vi "Set 2D Next Vector_IS_BAK.vi"(0 "Coordinate System":u16(ring) items=["Cartesian", "Polar"], 1 "Magnetic Field Units":u16(ring) items=["kG", "Tesla"], 2 "Input Vector":string[](array[string]), 3 "User defined Ramp Rate (T/min)":dbl format="%.3f", 4 "Magnitude Limit (kG)":dbl format="%.3f", 5 "Y-Axis Communications Config":T3={"GPIB address"=22, "GPIB bus"=0, "connection ID"=refnum, "IP"="192.168.2.200", "Active Comm Interface"=0, "Serial Port"="", "Programmer Type"=0} {"Programmer Type" items=["Model 430", "Model 420"]; "Active Comm Interface" items=["TCP/IP (Model 430 Only)", "RS232", "IEEE488"]}, 6 "Tolerance (mT)":dbl=0.2 format="%#_13g", 7 "Z-Axis Communications Config":T3={"GPIB address"=22, "GPIB bus"=0, "connection ID"=refnum, "IP"="192.168.2.200", "Active Comm Interface"=0, "Serial Port"="", "Programmer Type"=0} {"Programmer Type" items=["Model 430", "Model 420"]; "Active Comm Interface" items=["TCP/IP (Model 430 Only)", "RS232", "IEEE488"]}, 9 "Tolerance (deg)":dbl=0.1 format="%#_13g", 10 "User defined Ramp Rate (T/min)":bool, 13 "Max Ramp Rate - Y Axis (A/s)":dbl format="%.3f", 14 "error in":T2, 15 "Max Ramp Rate - Z Axis (A/s)":dbl format="%.3f") -> (8 "Current Magnetic\nField\n(430 TCP reading)":T1 {"phi (deg)" format="%#_3g"}, 11 "Y-Axis Ramp Rate (T/min)":dbl format="%.3f", 12 "Within Limits?":bool, 16 "Ramp Rate along Vector (T/min)":dbl, 17 "Z-Axis Ramp Rate (T/min)":dbl format="%.3f", 18 "All Instruments Responded?":bool, 19 "error out":T2)   [LabVIEW 2013]
uses:
  AMI reading polar field.ctl
  app/app global state actions.ctl
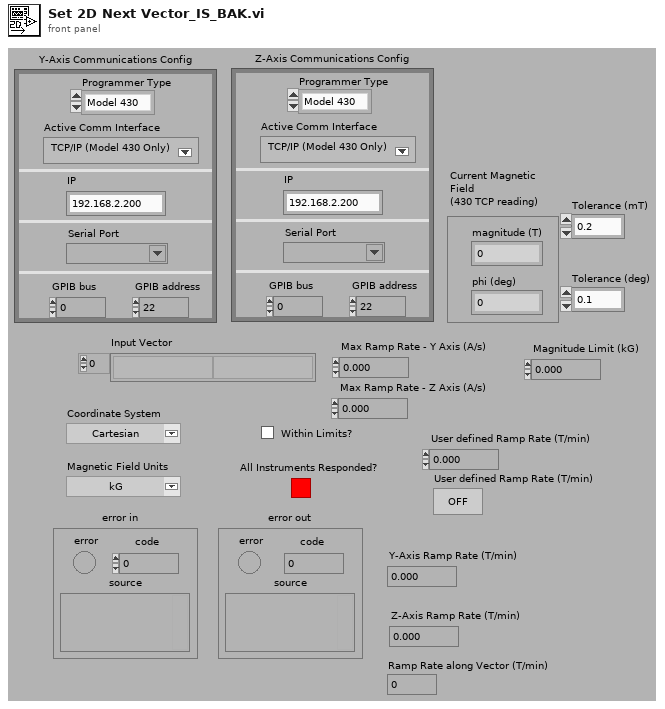
[diagram p1: front panel]
types:
  T1 = typedef "AMI reading polar field.ctl" = cluster{"magnitude (T)":dbl, "phi (deg)":dbl}
  T2 = cluster{"error":bool, "code":i32, "source":string}
  T3 = cluster{"GPIB address":i16, "GPIB bus":i16, "connection ID":refnum<k5>, "IP":string, "Active Comm Interface":u16, "Serial Port":refnum<visa-resource-name>, "Programmer Type":u16}
  T4 = typedef "app global state actions.ctl" = enum16{"get cluster", "set cluster", "set current sweep", "set field value", "set 430 TCP reading", "set ramping", "set sweeping", "append log", "clear log", "set finished"}
  T5 = cluster{"Radial (r) Field (T)":dbl, "phi (deg)":dbl}
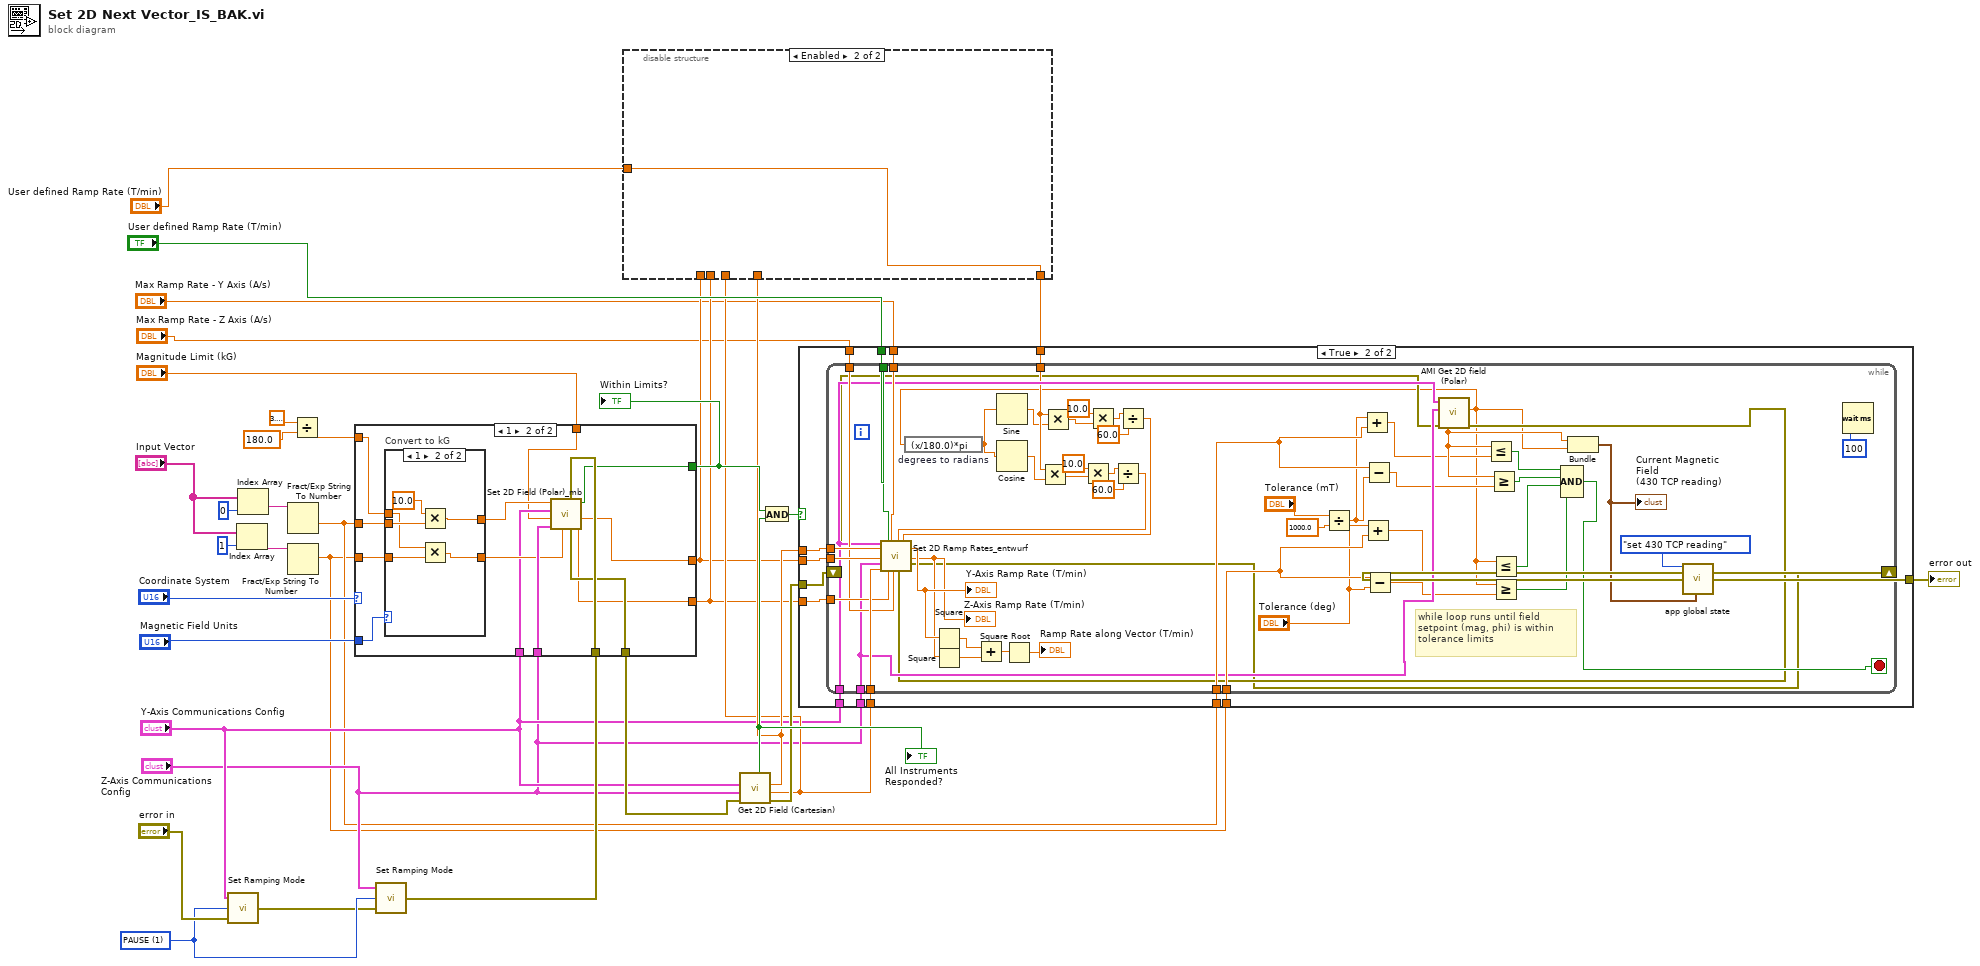
[diagram p0: block diagram]
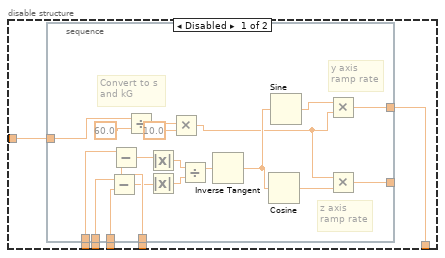
[diagram p2: hidden frame]
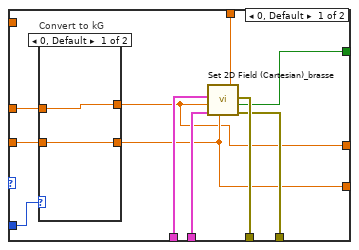
[diagram p4: hidden frame]
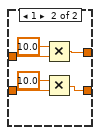
[diagram p5: hidden frame]
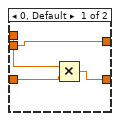
[diagram p6: hidden frame]
diagram:
  w21 = u16 1 items=["RAMP", "PAUSE", "MANUAL UP", "MANUAL DOWN", "ZERO"] ("Ramping Mode")
  n1 = call <userlib>:"Set Ramping Mode.vi"("error in"="error in", "Ramping Mode"=w21, "Communications Config"="Y-Axis Communications Config") -> ("error out"=w5:T2)
  n2 = Index Array(array="Input Vector", index=1 ("Index")) -> (element=w30:string)
  n3 = Index Array(array="Input Vector", index=0 ("Index")) -> (element=w31:string)
  n4 = Fract/Exp String To Number(string=w31) -> (number=w2:dbl)  [unwired: 3 in, 1 out]
  n5 = Fract/Exp String To Number(string=w30) -> (number=w1:dbl)  [unwired: 3 in, 1 out]
  n6 = Divide(x=3.141592653589793, y=180.0) -> (x/y=w15:dbl)
  n7 = call <userlib>:"Set Ramping Mode.vi"("error in"=w5, "Ramping Mode"=w21, "Communications Config"="Z-Axis Communications Config") -> ("error out"=w20:T2)
  n8 = case shown="1" "Coordinate System" {
    tunnel: "Magnetic Field Units" -> [w45 w67]
    tunnel: w2 -> [w44 w66]
    tunnel: w1 -> [w43 w65]
    tunnel: "Y-Axis Communications Config" -> [w42 w56]
    tunnel: "Z-Axis Communications Config" -> [w41 w62]
    tunnel: w20 -> [w40 w63]
    tunnel: [w39 w59] -> w28
    tunnel: [w38 w60] -> w19
    tunnel: [w37 w57] -> w10
    tunnel: [w36 w58] -> w9
    tunnel: w15 -> [_ w64]
    tunnel: "Magnitude Limit (kG)" -> [w35 w54]
    frame 0, Default {
      n9 = case "Convert to kG" shown="0, Default" w45 {
        tunnel: w44 -> [w47 w51]
        tunnel: w43 -> [w46 w50]
        tunnel: [w47 w49] -> w36
        tunnel: [w46 w48] -> w37
        frame 0, Default {
        }
        frame 1 {
          n10 = Multiply(x=10.0, y=w51) -> (x*y=w49:dbl)
          n11 = Multiply(x=10.0, y=w50) -> (x*y=w48:dbl)
        }
      }
      n12 = call <userlib>:"Set 2D Field (Cartesian)_brasse.vi"("error in"=w40, "Magnitude Limit (kG)"=w35, "Z-Axis Field (kG)"=w37, "Z-Axis Communications Config"=w41, "Y-Axis Field (kG)"=w36, "Y-Axis Communications Config"=w42) -> ("error out"=w38:T2, "Within Limits?"=w39:bool)  [unwired: 2 in]
    }
    frame 1 {
      n13 = case "Convert to kG" shown="1" w67 {
        tunnel: w66 -> [w70 w77]
        tunnel: w65 -> [w69 w76]
        tunnel: [w70 w75] -> w55
        tunnel: [w68 w74] -> w61
        tunnel: w64 -> [w71 w73]
        frame 0, Default {
          n14 = Multiply(x=w71, y=w69) -> (x*y=w68:dbl)
        }
        frame 1 {
          n15 = Multiply(x=10.0, y=w77) -> (x*y=w75:dbl)
          n16 = Multiply(x=w73, y=w76) -> (x*y=w74:dbl)
        }
      }
      n17 = call <userlib>:"Set 2D Field (Polar)_mb.vi"("error in"=w63, "f (radians)"=w61, "Z-Axis Communications Config"=w62, "Magnitude Limit (kG)"=w54, "Y-Axis Communications Config"=w56, "Field Magnitude r (kG)"=w55) -> ("Z-Axis Field (kG) out"=w57:dbl, "Y-Axis Field (kG)"=w58:dbl, "Within Limits?"=w59:bool, "error out"=w60:T2)  [unwired: 2 in]
    }
  }
  "Within Limits?" <- w28
  n18 = call <userlib>:"Get 2D Field (Cartesian).vi"("Y-Axis Communications Config"="Y-Axis Communications Config", "Z-Axis Communications Config"="Z-Axis Communications Config", "error in"=w19) -> ("All Instruments Responded?"=w26:bool, "Y-Axis Field (kG)"=w12:dbl, "Z-Axis Field (kG)"=w11:dbl, "error out"=w25:T2)  [unwired: 2 in]
  "All Instruments Responded?" <- w26
  n19 = disable-structure shown="Enabled" {
    disable-tunnel: "User defined Ramp Rate (T/min)" -> [w84 w104]
    disable-tunnel: [w82 w104] -> w14
    disable-tunnel: w12 -> [w81 _]
    disable-tunnel: w11 -> [w80 _]
    disable-tunnel: w10 -> [w79 _]
    disable-tunnel: w9 -> [w78 _]
    frame Disabled {
      n20 = stacked-sequence {
        tunnel: w84 -> [w99]
        tunnel: [w94] -> w82
        tunnel: [w93] -> w83
        tunnel: w81 -> [w92]
        tunnel: w80 -> [w91]
        tunnel: w79 -> [w86]
        tunnel: w78 -> [w85]
        frame #0 {
          # "y axis \nramp rate"
          # "z axis \nramp rate"
          # "Convert to s\nand kG"
          n21 = Subtract(x=w86, y=w91) -> (x-y=w89:dbl)
          n22 = Subtract(x=w85, y=w92) -> (x-y=w90:dbl)
          n23 = Divide(x=w99, y=60.0) -> (x/y=w97:dbl)
          n24 = Absolute Value(x=w90) -> (abs(x)=w87:dbl)
          n25 = Absolute Value(x=w89) -> (abs(x)=w88:dbl)
          n26 = Multiply(x=w97, y=10.0) -> (x*y=w95:dbl)
          n27 = Divide(x=w87, y=w88) -> (x/y=w103:dbl)
          n28 = Inverse Tangent(1:w103) -> (0:w102:dbl)
          n29 = Cosine(x=w102) -> (cos(x)=w100:dbl)
          n30 = Sine(x=w102) -> (sin(x)=w101:dbl)
          n31 = Multiply(x=w101, y=w95) -> (x*y=w94:dbl)
          n32 = Multiply(x=w95, y=w100) -> (x*y=w93:dbl)
        }
      }
    }
    frame Enabled {
    }
  }
  n33 = And(x=w28, y=w26) -> (x .and. y?=w27:bool)
  n34 = case shown="True" w27 {
    tunnel: "Y-Axis Communications Config" -> [_ w119]
    tunnel: "Z-Axis Communications Config" -> [_ w118]
    tunnel: w12 -> [_ w117]
    tunnel: w11 -> [_ w116]
    tunnel: w10 -> [_ w115]
    tunnel: w9 -> [_ w114]
    tunnel: w25 -> [w105 w110]
    tunnel: [w105 w113] -> w6
    tunnel: w14 -> [_ w112]
    tunnel: "User defined Ramp Rate (T/min)" -> [_ w111]
    tunnel: "Max Ramp Rate - Y Axis (A/s)" -> [_ w109]
    tunnel: "Max Ramp Rate - Z Axis (A/s)" -> [_ w108]
    tunnel: w2 -> [_ w107]
    tunnel: w1 -> [_ w106]
    frame False {
    }
    frame True {
      n35 = while {
        tunnel: w119 -> [w155]
        tunnel: w118 -> [w154]
        tunnel: w117 -> [w171]
        tunnel: w116 -> [w170]
        tunnel: w115 -> [w169]
        tunnel: w114 -> [w168]
        tunnel: w112 -> [w153]
        tunnel: w111 -> [w167]
        shift-right: [w120] -> w113
        shift-left: w110 -> [w151]
        tunnel: w109 -> [w159]
        tunnel: w108 -> [w158]
        tunnel: w107 -> [w157]
        tunnel: w106 -> [w156]
        stop <- w152 stop-if-true
        # "while loop runs until field \nsetpoint (mag, phi) is within \ntolerance limits"
        n36 = Divide(x="Tolerance (mT)", y=1000.0) -> (x/y=w140:dbl)
        n37 = Add(x=w140, y=w157) -> (x+y=w138:dbl)
        n38 = Add(x="Tolerance (deg)", y=w156) -> (x+y=w136:dbl)
        n39 = Subtract(x=w157, y=w140) -> (x-y=w137:dbl)
        n40 = Subtract(x=w156, y="Tolerance (deg)") -> (x-y=w135:dbl)
        n41 = call "AMI Get 2D field (Polar).vi"("error in"=w151, "Z-Axis Communications Config"=w154, "Y-Axis Communications Config"=w155) -> ("error out"=w150:T2, "phi (deg)"=w134:dbl, "Radial (r) Field (T)"=w147:dbl)  [unwired: 6 in]
        n42 = expression code="(x/180.0)*pi" "degrees to radians"(w134) -> (w127:dbl)
        n43 = Sine(x=w127) -> (sin(x)=w129:dbl)
        n44 = Cosine(x=w127) -> (cos(x)=w128:dbl)
        n45 = Multiply(x=w153, y=w128) -> (x*y=w133:dbl)
        n46 = Multiply(x=w153, y=w129) -> (x*y=w123:dbl)
        n47 = Multiply(x=10.0, y=w133) -> (x*y=w131:dbl)
        n48 = Multiply(x=10.0, y=w123) -> (x*y=w125:dbl)
        n49 = Divide(x=w131, y=60.0 ("x")) -> (x/y=w121:dbl)
        n50 = Divide(x=w125, y=60.0 ("x")) -> (x/y=w122:dbl)
        n51 = call <userlib>:"Set 2D Ramp Rates_entwurf.vi"("Y-Axis Communications Config"=w155, "Y-Axis Field (kG)"=w171, "Next Y-Axis Field (kG)"=w168, "Z-Axis Communications Config"=w154, "Z-Axis Field (kG)"=w170, "User defined Ramp Rate (T/min)"=w167, "Next Z-Axis Field (kG)"=w169, "Max Ramp Rate - Y Axis (A/s)"=w159, "Max Ramp Rate - Z Axis (A/s)"=w158, "User defined Ramp Rate - Z Axis (kG/s)"=w121, "error in"=w150, "User defined Ramp Rate Y-Axis (kG/s)"=w122) -> ("Y-Axis Ramp Rate (T/min)"=w166:dbl, "Z-Axis Ramp Rate (T/min)"=w165:dbl, "error out"=w120:T2)  [unwired: 5 in]
        "Y-Axis Ramp Rate (T/min)" <- w166
        "Z-Axis Ramp Rate (T/min)" <- w165
        n52 = Square(x=w166) -> (x^2=w163:dbl)
        n53 = Square(x=w165) -> (x^2=w164:dbl)
        n54 = Add(x=w163, y=w164) -> (x+y=w162:dbl)
        n55 = Square Root(x=w162) -> (sqrt(x)=→"Ramp Rate along Vector (T/min)":dbl)
        n56 = Less Or Equal?(x=w147, y=w138) -> (x <= y?=w149:bool)
        n57 = Greater Or Equal?(x=w147, y=w137) -> (x >= y?=w148:bool)
        n58 = Less Or Equal?(x=w134, y=w136) -> (x <= y?=w146:bool)
        n59 = Greater Or Equal?(x=w134, y=w135) -> (x >= y?=w145:bool)
        n60 = Compound Arithmetic op=AND(w149, w148, w146, w145) -> (w152:bool)
        n61 = Bundle("Radial (r) Field (T)"=w147, "phi (deg)"=w134) -> (w143:T5)  [unwired: 1 in]
        "Current Magnetic\nField\n(430 TCP reading)" <- w143
        n62 = call "app global state.vi"("action"=app_global_state_actions."set 430 TCP reading" ("app global state actions"), "Current Magnetic Field\n(430 TCP reading)"=w143) -> ()  [unwired: 17 in, 1 out]
        n63 = Wait (ms)(milliseconds to wait=100) -> ()  [unwired: 1 out]
      }
    }
  }
  "error out" <- w6
